vi "DHE_GetObsParams.vi"() -> (1 "obs string":string, 2 "DHE_OBS":T1={"observer"="", "obstype"="", "exptime"=0.0, "coadds"=1, "fowler"=1, "nimages"=0, "display"=TRUE, "autowrite"=TRUE, "frames to write"={"subs"=FALSE, "reset"=FALSE, "exposed"=FALSE}, "frames to display"={"subs"=FALSE, "reset"=FALSE, "exposed"=FALSE}, "sur"=0} {"exptime" format="%.2f"})   [LabVIEW 2016]
uses:
  private/vis/DHE_Obs.ctl
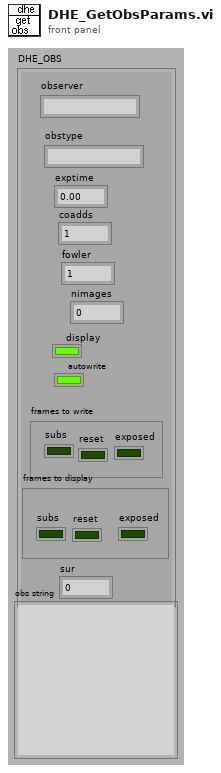
[diagram p1: front panel]
types:
  T1 = typedef "DHE_Obs.ctl" = cluster{"observer":string, "obstype":string, "exptime":dbl, "coadds":i32, "fowler":i32, "nimages":i32, "display":bool, "autowrite":bool, "frames to write":cluster{"subs":bool, "reset":bool, "exposed":bool}, "frames to display":cluster{"subs":bool, "reset":bool, "exposed":bool}, "sur":i32}
  T2 = typedef "DatabaseHand_RefNum.ctl" = refnum<vi>
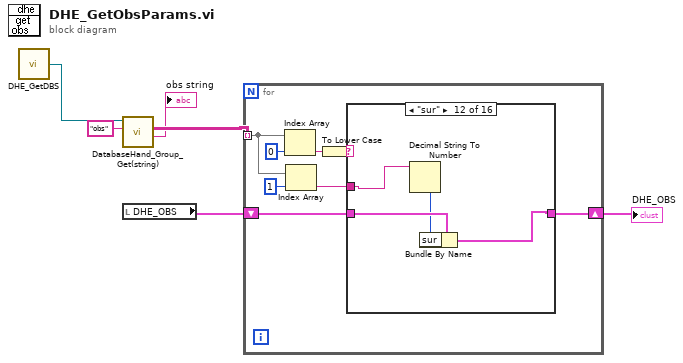
[diagram p0: block diagram]
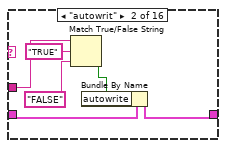
[diagram p3: hidden frame]
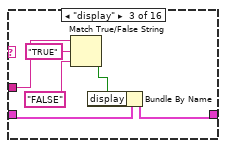
[diagram p4: hidden frame]
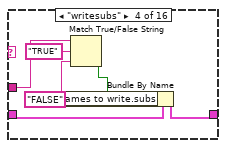
[diagram p5: hidden frame]
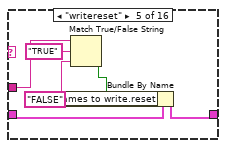
[diagram p6: hidden frame]
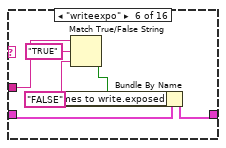
[diagram p7: hidden frame]
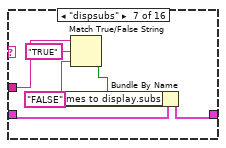
[diagram p8: hidden frame]
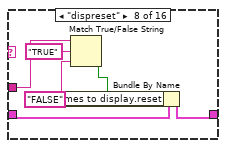
[diagram p9: hidden frame]
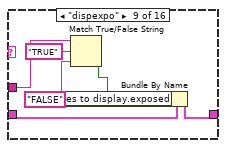
[diagram p10: hidden frame]
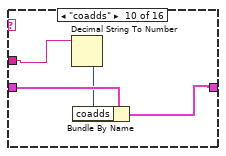
[diagram p11: hidden frame]
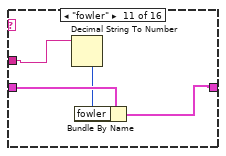
[diagram p12: hidden frame]
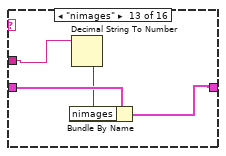
[diagram p13: hidden frame]
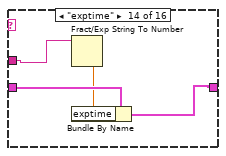
[diagram p14: hidden frame]
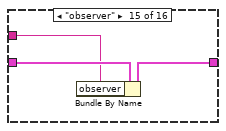
[diagram p15: hidden frame]
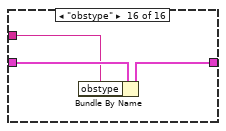
[diagram p16: hidden frame]
diagram:
  n1 = call "DHE_GetDBS.vi"() -> ("DHE_DBSRef"=w1:T2)  [unwired: 9 out]
  n2 = call "DatabaseHand_Group_Get(string).vi"("group"="obs", "Database RefNum in"=w1) -> ("group string"=→"obs string":string, "group array"=w5:string[][])  [unwired: 1 in, 7 out]
  n3 = local read "DHE_OBS"() -> (w4:T1)
  n4 = for {
    tunnel: w5 -> [w9] mode=indexing
    shift-right: [w11] -> w3
    shift-left: w4 -> [w12]
    n5 = Index Array(array=w9, index=0) -> (element=w13:string)
    n6 = Index Array(array=w9, index=1) -> (element=w8:string)
    n7 = To Lower Case(string=w13) -> (all lower case string=w7:string)
    n8 = case shown="\"sur\"" w7 {
      tunnel: w12 -> [w15 w21 w27 w33 w39 w45 w51 w57 w63 w67 w71 w75 w79 w83 w86 w89]
      tunnel: [w15 w20 w26 w32 w38 w44 w50 w56 w62 w66 w70 w74 w78 w82 w85 w88] -> w11
      tunnel: w8 -> [_ w19 w25 w31 w37 w43 w49 w55 w61 w65 w69 w73 w77 w81 w84 w87]
      frame Default {
      }
      frame "autowrit" {
        n9 = Match True/False String(2:"FALSE" ("false string"), 3:"TRUE" ("true string"), 4:w19) -> (0:w18:bool)  [unwired: 1 out]
        n10 = Bundle By Name(cluster=w21, "autowrite"=w18) -> (w20:T1)
      }
      frame "display" {
        n11 = Match True/False String(2:"FALSE" ("false string"), 3:"TRUE" ("true string"), 4:w25) -> (0:w24:bool)  [unwired: 1 out]
        n12 = Bundle By Name(cluster=w27, "display"=w24) -> (w26:T1)
      }
      frame "writesubs" {
        n13 = Match True/False String(2:"FALSE" ("false string"), 3:"TRUE" ("true string"), 4:w31) -> (0:w30:bool)  [unwired: 1 out]
        n14 = Bundle By Name(cluster=w33, "frames to write.subs"=w30) -> (w32:T1)
      }
      frame "writereset" {
        n15 = Match True/False String(2:"FALSE" ("false string"), 3:"TRUE" ("true string"), 4:w37) -> (0:w36:bool)  [unwired: 1 out]
        n16 = Bundle By Name(cluster=w39, "frames to write.reset"=w36) -> (w38:T1)
      }
      frame "writeexpo" {
        n17 = Match True/False String(2:"FALSE" ("false string"), 3:"TRUE" ("true string"), 4:w43) -> (0:w42:bool)  [unwired: 1 out]
        n18 = Bundle By Name(cluster=w45, "frames to write.exposed"=w42) -> (w44:T1)
      }
      frame "dispsubs" {
        n19 = Match True/False String(2:"FALSE" ("false string"), 3:"TRUE" ("true string"), 4:w49) -> (0:w48:bool)  [unwired: 1 out]
        n20 = Bundle By Name(cluster=w51, "frames to display.subs"=w48) -> (w50:T1)
      }
      frame "dispreset" {
        n21 = Match True/False String(2:"FALSE" ("false string"), 3:"TRUE" ("true string"), 4:w55) -> (0:w54:bool)  [unwired: 1 out]
        n22 = Bundle By Name(cluster=w57, "frames to display.reset"=w54) -> (w56:T1)
      }
      frame "dispexpo" {
        n23 = Match True/False String(2:"FALSE" ("false string"), 3:"TRUE" ("true string"), 4:w61) -> (0:w60:bool)  [unwired: 1 out]
        n24 = Bundle By Name(cluster=w63, "frames to display.exposed"=w60) -> (w62:T1)
      }
      frame "coadds" {
        n25 = Decimal String To Number(string=w65) -> (number=w64:i32)  [unwired: 3 out]
        n26 = Bundle By Name(cluster=w67, "coadds"=w64) -> (w66:T1)
      }
      frame "fowler" {
        n27 = Decimal String To Number(string=w69) -> (number=w68:i32)  [unwired: 3 out]
        n28 = Bundle By Name(cluster=w71, "fowler"=w68) -> (w70:T1)
      }
      frame "sur" {
        n29 = Decimal String To Number(string=w73) -> (number=w72:i32)  [unwired: 3 out]
        n30 = Bundle By Name(cluster=w75, "sur"=w72) -> (w74:T1)
      }
      frame "nimages" {
        n31 = Decimal String To Number(string=w77) -> (number=w76:i32)  [unwired: 3 out]
        n32 = Bundle By Name(cluster=w79, "nimages"=w76) -> (w78:T1)
      }
      frame "exptime" {
        n33 = Fract/Exp String To Number(string=w81) -> (number=w80:dbl)  [unwired: 4 out]
        n34 = Bundle By Name(cluster=w83, "exptime"=w80) -> (w82:T1)
      }
      frame "observer" {
        n35 = Bundle By Name(cluster=w86, "observer"=w84) -> (w85:T1)
      }
      frame "obstype" {
        n36 = Bundle By Name(cluster=w89, "obstype"=w87) -> (w88:T1)
      }
    }
  }
  "DHE_OBS" <- w3
